vi "Ring Buffer CH3 long.vi"(9 "Index":i32, 10 "Profiles to Average":i32, 11 "Input Array":dbl[](array[numeric])) -> (1 "AvgArray":dbl[](array[numeric]), 3 "RingBufferOut":dbl[][](array[numeric]))   [LabVIEW 2012]
panel:
  out "RingArraySize":dbl[](array[numeric])
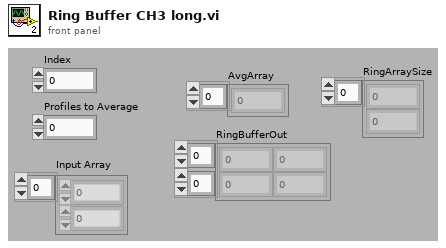
[diagram p1: front panel]
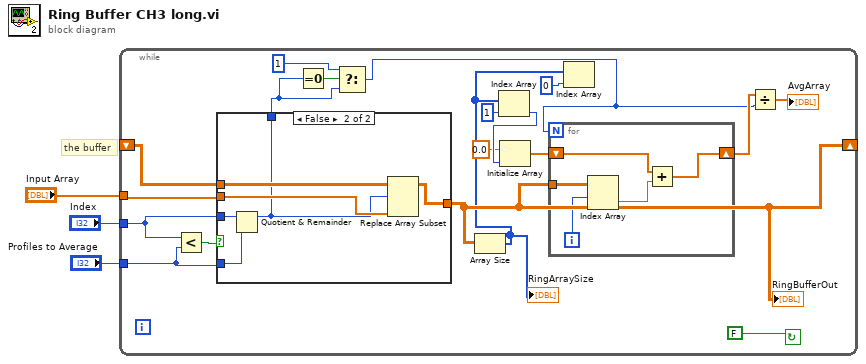
[diagram p0: block diagram]
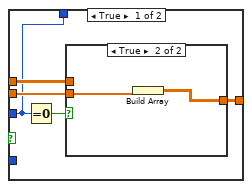
[diagram p2: hidden frame]
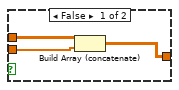
[diagram p3: hidden frame]
diagram:
  # "the buffer"
  n1 = while {
    shift-right: [w14] -> _
    shift-left: _ -> [w17]
    tunnel: "Profiles to Average" -> [w20]
    tunnel: "Index" -> [w19]
    tunnel: "Input Array" -> [w18]
    stop <- FALSE ("stop") continue-if-true
    n2 = Less?(x=w19, y=w20) -> (x < y?=w21:bool)
    n3 = case shown="False" w21 {
      tunnel: w19 -> [w28 w43]
      tunnel: [w29 w39] -> w14
      tunnel: w20 -> [_ w42]
      tunnel: w18 -> [w30 w40]
      tunnel: w17 -> [w31 w41]
      tunnel: [w28 w38] -> w5
      frame True {
        n4 = Equal To 0?(x=w28) -> (x = 0?=w32:bool)
        n5 = case shown="True" w32 {
          tunnel: [w33 w37] -> w29
          tunnel: w31 -> [w35 _]
          tunnel: w30 -> [w34 w36]
          frame False {
            n6 = Build Array (concatenate)(w35, w34) -> (w33:dbl[][])
          }
          frame True {
            n7 = Build Array(w36) -> (w37:dbl[][])
          }
        }
      }
      frame False {
        n8 = Quotient & Remainder(x=w43, y=w42) -> (x-y*floor(x/y)=w38:i32)  [unwired: 1 out]
        n9 = Replace Array Subset(array=w41, new element=w40, index (row)=w38) -> (w39:dbl[][])  [unwired: 1 in]
      }
    }
    "RingBufferOut" <- w14
    n10 = Equal To 0?(x=w5) -> (x = 0?=w7:bool)
    n11 = Select(t=1, s=w7, f=w5) -> (s? t:f=w4:i32)
    n12 = Array Size(array=w14) -> (size(s)=w8:i32[])
    "RingArraySize" <- w8
    n13 = Index Array(array=w8, index=1) -> (element=w13:i32)
    n14 = Initialize Array(0.0, w13) -> (w11:dbl[])
    n15 = for {
      N: w4 -> [_]
      tunnel: w14 -> [w27]
      shift-right: [w23] -> w10
      shift-left: w11 -> [w24]
      i -> [w26]
      n16 = Index Array(array=w27, index (row)=w26) -> (element=w25:dbl[])  [unwired: 1 in]
      n17 = Add(x=w24, y=w25) -> (x+y=w23:dbl[])
    }
    n18 = Index Array(array=w8, index=0) -> ()  [unwired: 1 out]
    n19 = Divide(x=w10, y=w4) -> (x/y=→"AvgArray":dbl[])
  }
